vi "I2C Message Buffer - Check.vi"(8 "error in (no error)":errorcluster) -> (0 "error out":errorcluster, 3 "# elements in queue":i32)   [LabVIEW 2025, in "I2C Bus Monitor.lvclass"]
uses:
  I2C Bus Monitor.lvclass
  I2C Bus Monitor.lvclass/I2C Bus Monitor.ctl
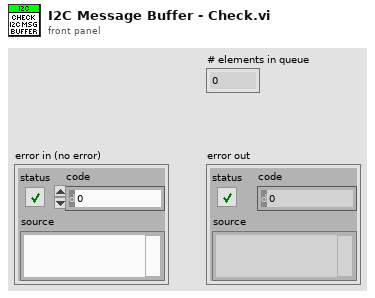
[diagram p1: front panel]
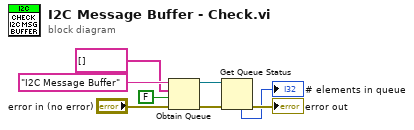
[diagram p0: block diagram]
diagram:
  n1 = Obtain Queue(name (unnamed)="I2C Message Buffer", element data type=string[] [] ("I2C Messages"), create if not found? (T)=FALSE, error in (no error)="error in (no error)") -> (queue out=w2:refnum<queue>, error out=w5:errorcluster)  [unwired: 1 in, 1 out]
  n2 = Get Queue Status(queue=w2, error in (no error)=w5) -> (error out=→"error out":errorcluster, # elements in queue=→"# elements in queue":i32)  [unwired: 1 in, 6 out]
